vi "Terminla_GearSystem_Work_Condition.vi"(11 "齿轮子系统监测参数":T1) -> (3 "达到工作条件":bool)   [LabVIEW 2014]
uses:
  Work_Condition.vi
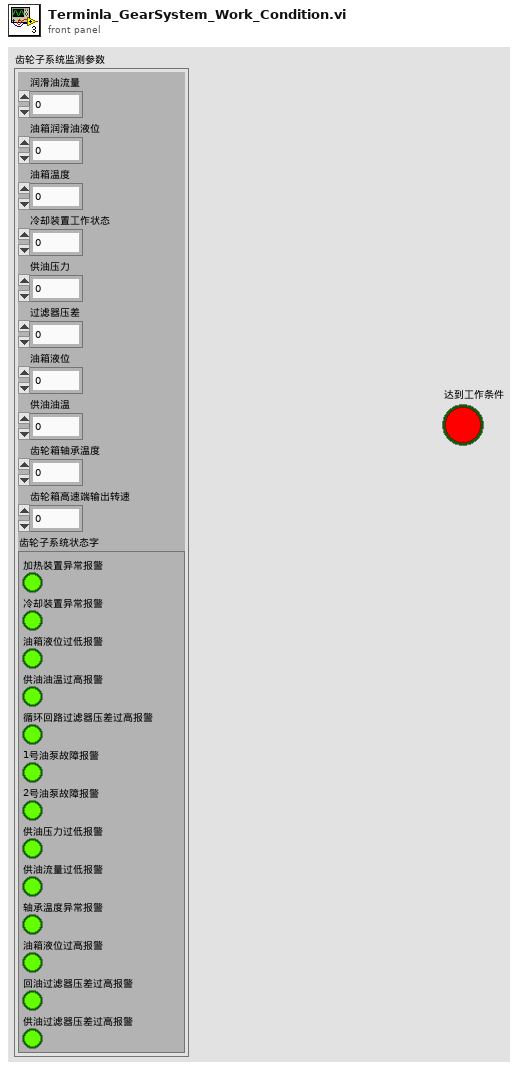
[diagram p1: front panel]
types:
  T1 = cluster{"润滑油流量":u16, "油箱润滑油液位":u16, "油箱温度":u16, "冷却装置工作状态":u16, "供油压力":u16, "过滤器压差":u16, "油箱液位":u16, "供油油温":u16, "齿轮箱轴承温度":u16, "齿轮箱高速端输出转速":u16, "齿轮子系统状态字":cluster{"加热装置异常报警":bool, "冷却装置异常报警":bool, "油箱液位过低报警":bool, "供油油温过高报警":bool, "循环回路过滤器压差过高报警":bool, "1号油泵故障报警":bool, "2号油泵故障报警":bool, "供油压力过低报警":bool, "供油流量过低报警":bool, "轴承温度异常报警":bool, "油箱液位过高报警":bool, "回油过滤器压差过高报警":bool, "供油过滤器压差过高报警":bool}}
  T2 = cluster{"加热装置异常报警":bool, "冷却装置异常报警":bool, "油箱液位过低报警":bool, "供油油温过高报警":bool, "循环回路过滤器压差过高报警":bool, "1号油泵故障报警":bool, "2号油泵故障报警":bool, "供油压力过低报警":bool, "供油流量过低报警":bool, "轴承温度异常报警":bool, "油箱液位过高报警":bool, "回油过滤器压差过高报警":bool, "供油过滤器压差过高报警":bool}
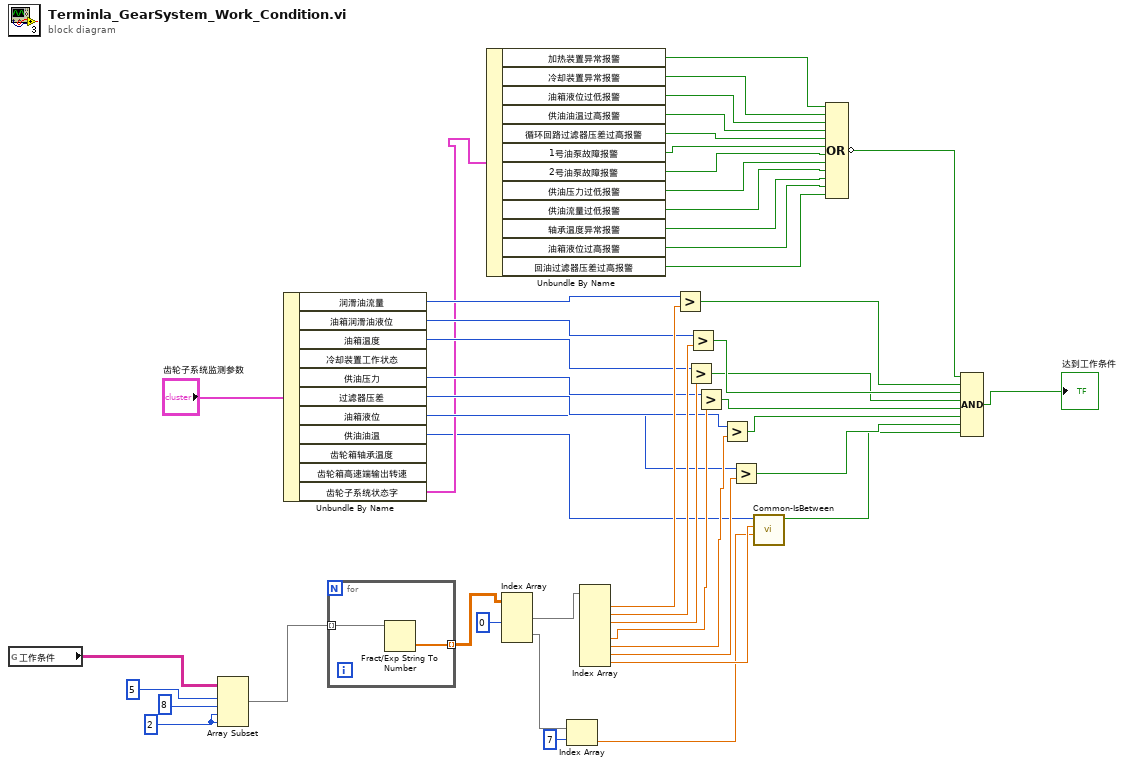
[diagram p0: block diagram]
diagram:
  w48 = 2
  n1 = global read "Work_Condition.vi" "工作条件"() -> (w6:string[][])
  n2 = Array Subset(array=w6, index (row)=5, length (row)=8, index (col)=w48, length (col)=w48) -> (w47:string[][])
  n3 = Unbundle By Name("齿轮子系统监测参数") -> ("润滑油流量"=w42:u16, "油箱润滑油液位"=w40:u16, "油箱温度"=w38:u16, "供油压力"=w36:u16, "过滤器压差"=w34:u16, "油箱液位"=w32:u16, "供油油温"=w3:u16, "齿轮子系统状态字"=w21:T2)  [unwired: 3 out]
  n4 = for {
    tunnel: w47 -> [w50] mode=indexing
    tunnel: [w49] -> w46 mode=indexing
    n5 = Fract/Exp String To Number(string=w50) -> (number=w49:dbl[])  [unwired: 3 in, 1 out]
  }
  n6 = Unbundle By Name(w21) -> ("加热装置异常报警"=w20:bool, "冷却装置异常报警"=w19:bool, "油箱液位过低报警"=w18:bool, "供油油温过高报警"=w17:bool, "循环回路过滤器压差过高报警"=w16:bool, "1号油泵故障报警"=w15:bool, "2号油泵故障报警"=w14:bool, "供油压力过低报警"=w13:bool, "供油流量过低报警"=w12:bool, "轴承温度异常报警"=w11:bool, "油箱液位过高报警"=w10:bool, "回油过滤器压差过高报警"=w9:bool)
  n7 = Index Array(array=w46, index (col) #1=0) -> (element #1=w44:dbl[], element #2=w43:dbl[])  [unwired: 3 in]
  n8 = Index Array(array=w43, index=7) -> (element=w1:dbl)
  n9 = Index Array(array=w44) -> (element #1=w41:dbl, element #2=w39:dbl, element #3=w37:dbl, element #5=w35:dbl, element #6=w33:dbl, element #7=w31:dbl, element #8=w2:dbl)  [unwired: 8 in, 1 out]
  n10 = Greater?(x=w42, y=w41) -> (0:w29:bool)
  n11 = Greater?(x=w38, y=w37) -> (0:w27:bool)
  n12 = Greater?(x=w40, y=w39) -> (0:w28:bool)
  n13 = Greater?(x=w36, y=w35) -> (0:w26:bool)
  n14 = Greater?(x=w34, y=w33) -> (0:w25:bool)
  n15 = Greater?(x=w32, y=w31) -> (0:w24:bool)
  n16 = call "Common-IsBetween.vi"("比例(0.1)"=w1, "基数"=w2, "x"=w3) -> ("范围内？"=w23:bool)  [unwired: 8 in]
  n17 = Compound Arithmetic op=OR(w20, w19, w18, w17, w16, w15, w14, w13, w12, w11, w10, w9) -> (invert w8:bool)
  n18 = Compound Arithmetic op=AND(w8, w29, w28, w27, w26, w25, w24, w23) -> (→"达到工作条件":bool)
